vi "Read NET_ByteArrayContent.vi"(8 "error in (no error)":errorcluster, 11 "HttpContent_String in":refnum<class "HttpContent_ByteArray.lvclass">) -> (0 "error out":errorcluster, 2 "NET_ByteArrayContent":refnum<k24>, 3 "HttpContent_String out":refnum<class "HttpContent_ByteArray.lvclass">)   [LabVIEW 2018, in "HttpClient_NET.lvlib" / "HttpContent_ByteArray.lvclass"]
uses:
  HttpContent_ByteArray.lvclass
  C:/Viviota/Projects/R&D/LabVIEW_HTTP_REST_NET/HttpContent/HttpContent.lvclass
  System.Net.Http
  HttpContent/HttpContent.lvclass/HttpContent.ctl
  HttpContent/HttpContent.lvclass
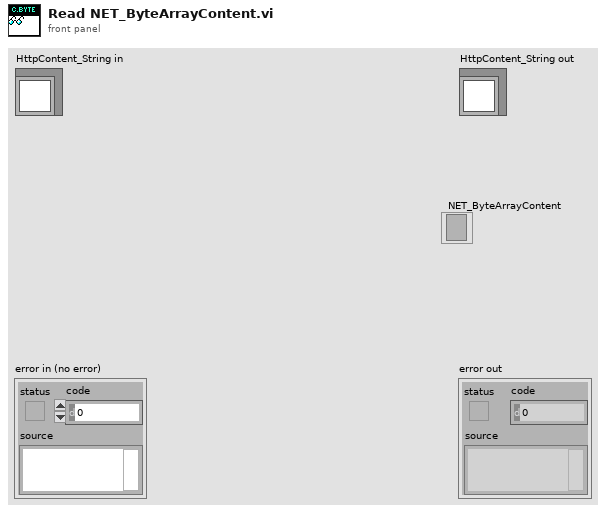
[diagram p1: front panel]
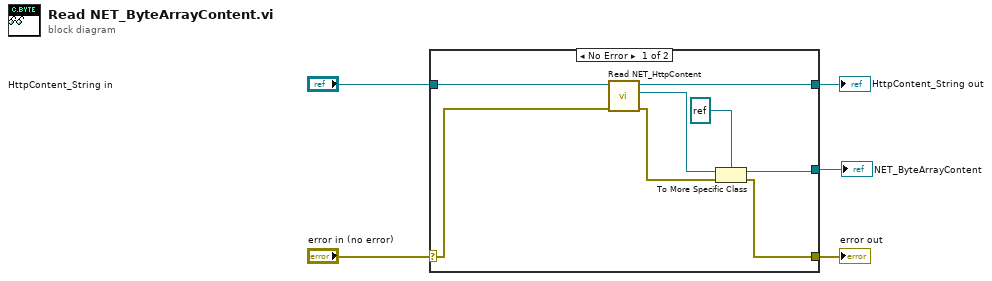
[diagram p0: block diagram]
diagram:
  n1 = case shown="No Error" "error in (no error)" {
    selector: "error in (no error)" -> [w10 w14]
    tunnel: [w8 w14] -> w4
    tunnel: [w12 w15] -> w2
    tunnel: "HttpContent_String in" -> [w13 w15]
    tunnel: [w11 _] -> w1
    frame No Error {
      n2 = call "Read NET_HttpContent.vi"("error in (no error)"=w10, "HttpContent in"=w13) -> ("error out"=w9:errorcluster, "NET_HttpContent"=w7:refnum<k24>, "HttpContent out"=w12:refnum<class "HttpContent_ByteArray.lvclass">)  [unwired: 7 in]
      n3 = To More Specific Class(target class=refnum<k24> refnum ("NET_ByteArrayContent"), reference=w7, error in=w9) -> (specific class reference=w11:refnum<k24>, error out=w8:errorcluster)
    }
    frame Error {
    }
  }
  "error out" <- w4
  "HttpContent_String out" <- w2
  "NET_ByteArrayContent" <- w1
